vi "Process Rising Edge.vi"(6 "edge number (1)":i32=1 min=1, 8 "error in":errorcluster, 10 "PulseAnalysis in":T1, 11 "ChannelData in":waveform(dbl)) -> (0 "error out":errorcluster, 2 "PulseAnalysis out":T1, 3 "ChannelData Out":waveform(dbl))   [LabVIEW 2019, in "Variant Parser.lvlib" / "WaveformProcessor.lvclass"]
uses:
  Library/WaveformProcessor.lvclass
  Custom Controls/Pulse Analysis.ctl
  <vilib>/measure/mascope.llb/Transition Measurements 1 chan.vi
  <vilib>/measure/NI_MAPro.lvlib
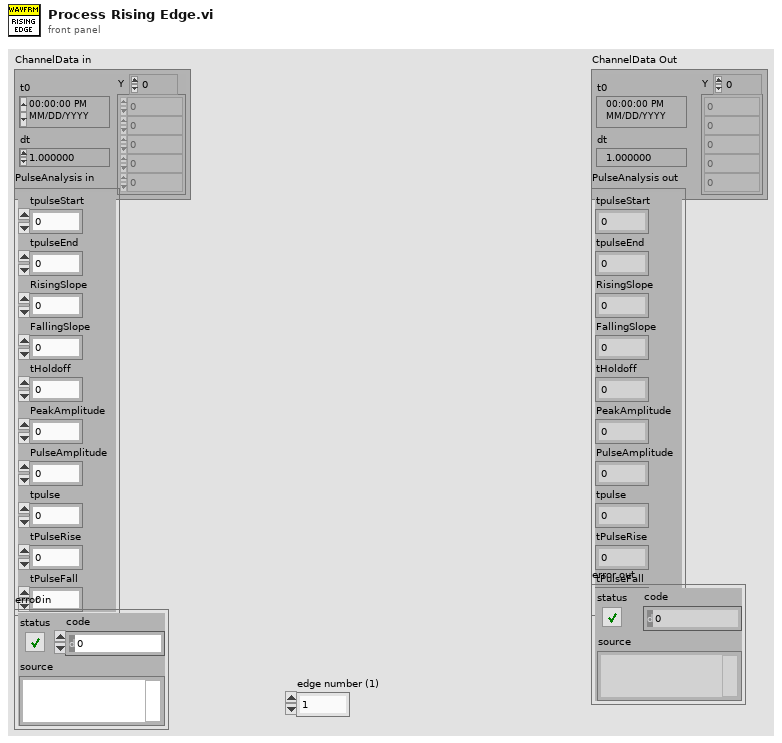
[diagram p1: front panel]
types:
  T1 = typedef "Variant Parser.lvlib/WaveformProcessor.lvclass/Pulse Analysis.ctl" = cluster{"tpulseStart":dbl, "tpulseEnd":dbl, "RisingSlope":dbl, "FallingSlope":dbl, "tHoldoff":dbl, "PeakAmplitude":dbl, "PulseAmplitude":dbl, "tpulse":dbl, "tPulseRise":dbl, "tPulseFall":dbl}
  T2 = cluster{"start time":dbl, "end time":dbl, "ref levels":cluster{"high ref level":dbl, "mid ref level":dbl, "low ref level":dbl, "ref units":u16}}
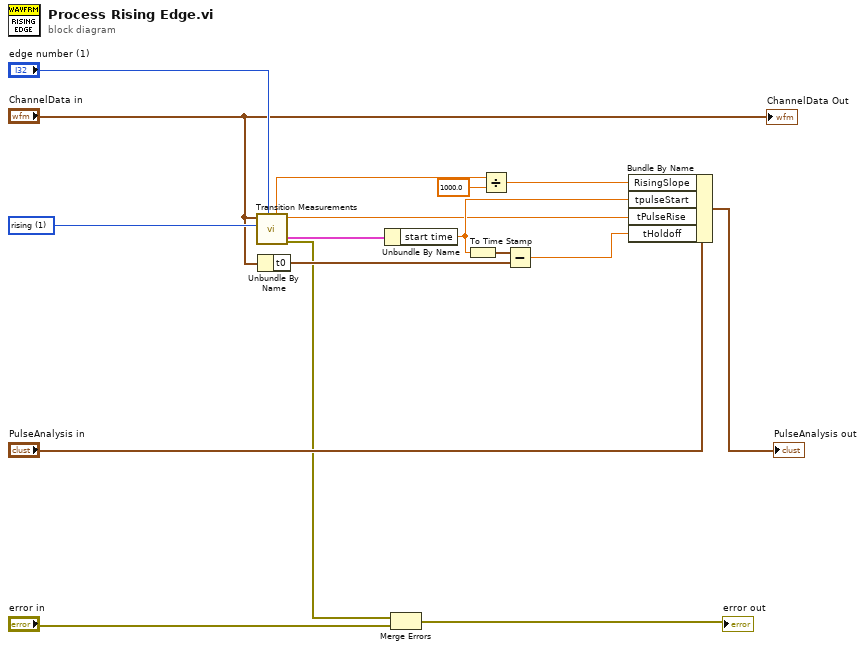
[diagram p0: block diagram]
diagram:
  w17 = u16 1 items=["falling", "rising"] ("polarity (rising)")
  n1 = call-poly <vilib>:"Transition Measurements.vi"("edge number (1)"="edge number (1)", "polarity (rising)"=w17, "signal in"="ChannelData in") -> ("error out"=w2:errorcluster, "transition duration"=w1:dbl, "measurement info"=w11:T2, "slope"=w14:dbl)  [unwired: 3 in, 2 out]
  n2 = Unbundle By Name("ChannelData in") -> ("t0"=w7:timestamp)
  n3 = Unbundle By Name(w11) -> ("start time"=w4:dbl)
  n4 = Merge Errors(w2, "error in") -> (→"error out":errorcluster)
  n5 = To Time Stamp(1:w4) -> (0:w6:timestamp)
  n6 = Divide(x=w14, y=1000.0) -> (x/y=w12:dbl)
  n7 = Subtract(x=w6, y=w7) -> (x-y=w5:dbl)
  n8 = Bundle By Name(cluster="PulseAnalysis in", "RisingSlope"=w12, "tpulseStart"=w4, "tPulseRise"=w1, "tHoldoff"=w5) -> (→"PulseAnalysis out":T1)
  "ChannelData Out" <- "ChannelData in"
